vi "Fetch QD Functions From Database.vi"(8 "error in (no error)":errorcluster, 10 "Keyword(\"\")":string, 11 "ToolLauncher in":refnum<class "ScriptDialog.lvclass">) -> (0 "error out":errorcluster, 2 "QDFunctionsData":variant[][](array[variant]), 3 "ToolLauncher out":refnum<class "ScriptDialog.lvclass">)   [LabVIEW 2015, in "ScriptDialog.lvclass"]
uses:
  ScriptDialog.lvclass
  ScriptDialog.lvclass/ScriptDialog.ctl
  _Database/Implements/ScriptDatabase.lvclass/ScriptDatabase.ctl
  _Database/Ancestor/DatabaseAPI.lvclass
  _Database/Implements/ScriptDatabase.lvclass
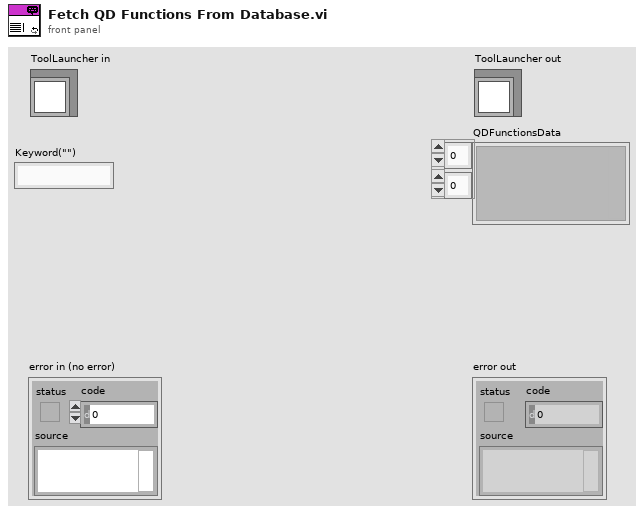
[diagram p1: front panel]
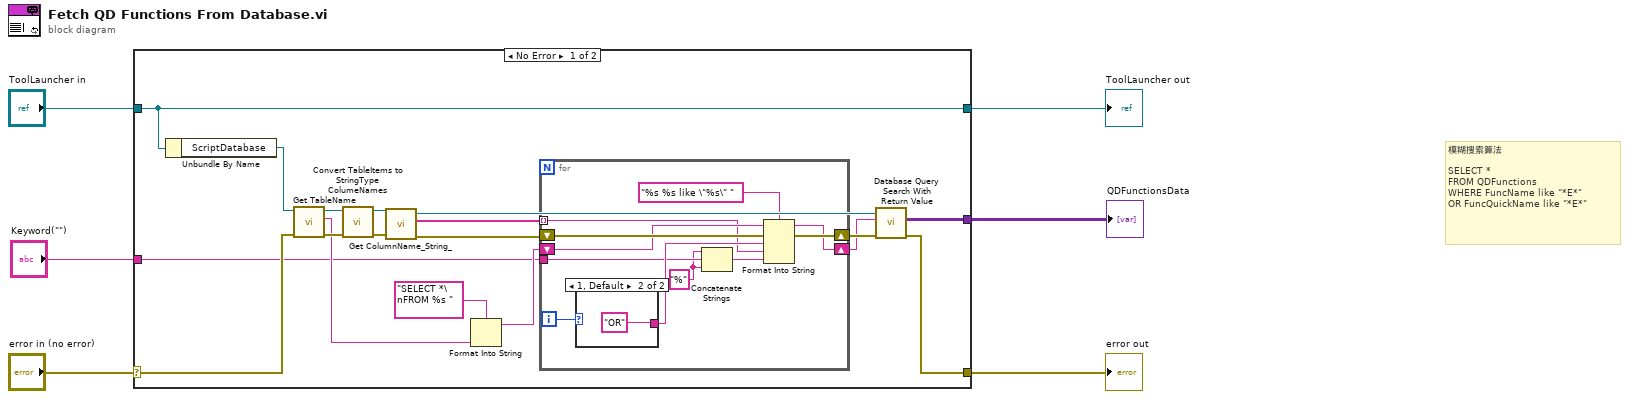
[diagram p0: block diagram]
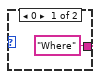
[diagram p2: hidden frame]
diagram:
  # "模糊搜索算法\n\nSELECT *\nFROM QDFunctions\nWHERE FuncName like \"*E*\" \nOR FuncQuickName like \"*E*\""
  n1 = case shown="No Error" "error in (no error)" {
    selector: "error in (no error)" -> [w19 w39]
    tunnel: [w9 w39] -> w5
    tunnel: [w24 w38] -> w3
    tunnel: "ToolLauncher in" -> [w24 w38]
    tunnel: "Keyword(\"\")" -> [w12 _]
    tunnel: [w7 _] -> w1
    frame No Error {
      n2 = Unbundle By Name(w24) -> ("ScriptDatabase"=w20:refnum<class "ScriptDatabase.lvclass">)
      n3 = call "Get TableName.vi"("error in (no error)"=w19, "ScriptDatabase in"=w20) -> ("error out"=w17:errorcluster, "TableName"=w16:string, "ScriptDatabase out"=w18:refnum<class "ScriptDatabase.lvclass">)  [unwired: 7 in]
      n4 = call "Convert TableItems to StringType ColumeNames.vi"("error in (no error)"=w17, "ScriptDatabase in"=w18) -> ("error out"=w14:errorcluster, "ScriptDatabase out"=w15:refnum<class "ScriptDatabase.lvclass">)  [unwired: 8 in]
      n5 = call "Get ColumnName_String_.vi"("error in (no error)"=w14, "ScriptDatabase in"=w15) -> ("error out"=w22:errorcluster, "ColumnName<String>"=w23:string[], "ScriptDatabase out"=w10:refnum<class "ScriptDatabase.lvclass">)  [unwired: 7 in]
      n6 = Format Into String(format string="SELECT *\nFROM %s ", w16) -> (resulting string=w13:string)  [unwired: 2 in, 1 out]
      n7 = for {
        tunnel: w23 -> [w28] mode=indexing
        tunnel: w12 -> [w27]
        shift-right: [w31] -> w11
        shift-left: w22 -> [w32]
        shift-right: [w29] -> w8
        shift-left: w13 -> [w30]
        i -> [w35]
        w25 = "%"
        n8 = case shown="1, Default" w35 {
          tunnel: ["Where" "OR"] -> w33
          frame 0 {
          }
          frame 1, Default {
          }
        }
        n9 = Concatenate Strings(w25, w27, w25) -> (w26:string)
        n10 = Format Into String(format string="%s %s like \"%s\" ", initial string=w30, error in=w32, w33, w28, w26) -> (resulting string=w29:string, error out=w31:errorcluster)
      }
      n11 = call "Database Query Search With Return Value.vi"("error in (no error)"=w11, "SQL query"=w8, "object in"=w10) -> ("error out"=w9:errorcluster, "recordset data"=w7:variant[][])  [unwired: 5 in, 2 out]
    }
    frame Error {
    }
  }
  "error out" <- w5
  "ToolLauncher out" <- w3
  "QDFunctionsData" <- w1
